vi "Stack Demo.vi"() -> ()   [LabVIEW 2011]
uses:
  Stack.lvclass
panel:
  out "AAA":variant
  out "BBB":variant
  out "Items":variant[](array[variant])
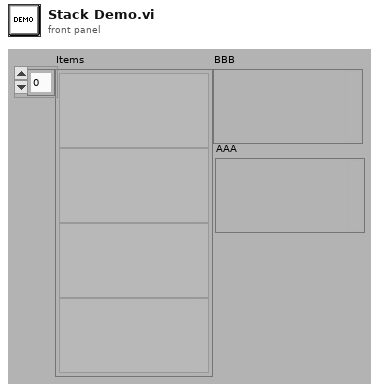
[diagram p1: front panel]
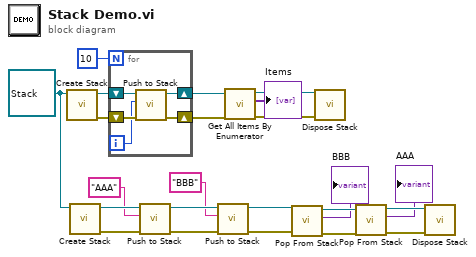
[diagram p0: block diagram]
diagram:
  w15 = refnum<class "Stack.lvclass"> refnum ("Stack.lvclass")
  n1 = call "Create Stack.vi"("Stack 输入"=w15) -> ("error out"=w21:errorcluster, "Stack 输出"=w22:refnum<class "Stack.lvclass">)  [unwired: 9 in]
  n2 = call "Create Stack.vi"("Stack 输入"=w15) -> ("error out"=w12:errorcluster, "Stack 输出"=w14:refnum<class "Stack.lvclass">)  [unwired: 9 in]
  n3 = for {
    N: 10 -> [_]
    shift-right: [w26] -> w19
    shift-left: w22 -> [w28]
    shift-right: [w25] -> w20
    shift-left: w21 -> [w27]
    i -> [w24]
    n4 = call "Push to Stack.vi"("error in (no error)"=w27, "Element"=w24, "Stack 输入"=w28) -> ("error out"=w25:errorcluster, "Stack 输出"=w26:refnum<class "Stack.lvclass">)  [unwired: 7 in]
  }
  n5 = call "Push to Stack.vi"("error in (no error)"=w12, "Element"="AAA", "Stack 输入"=w14) -> ("error out"=w11:errorcluster, "Stack 输出"=w13:refnum<class "Stack.lvclass">)  [unwired: 7 in]
  n6 = call "Push to Stack.vi"("error in (no error)"=w11, "Element"="BBB", "Stack 输入"=w13) -> ("error out"=w7:errorcluster, "Stack 输出"=w8:refnum<class "Stack.lvclass">)  [unwired: 7 in]
  n7 = call "Get All Items By Enumerator.vi"("error in (no error)"=w20, "Stack 输入"=w19) -> ("error out"=w17:errorcluster, "Items"=→"Items":variant[], "Stack 输出"=w18:refnum<class "Stack.lvclass">)  [unwired: 7 in]
  n8 = call "Pop From Stack.vi"("error in (no error)"=w7, "Stack 输入"=w8) -> ("error out"=w5:errorcluster, "Element"=→"BBB":variant, "Stack 输出"=w6:refnum<class "Stack.lvclass">)  [unwired: 7 in]
  n9 = call "Dispose Stack.vi"("error in (no error)"=w17, "Stack 输入"=w18) -> ()  [unwired: 8 in, 2 out]
  n10 = call "Pop From Stack.vi"("error in (no error)"=w5, "Stack 输入"=w6) -> ("error out"=w3:errorcluster, "Element"=→"AAA":variant, "Stack 输出"=w4:refnum<class "Stack.lvclass">)  [unwired: 7 in]
  n11 = call "Dispose Stack.vi"("error in (no error)"=w3, "Stack 输入"=w4) -> ()  [unwired: 8 in, 2 out]
